vi "Create User Waveform.vi"(6 "Phase (0.0 deg)":dbl[](array[numeric])=[0.0, 0.0, 0.0, 0.0, 0.0, 0.0, 0.0, 0.0, 0.0, 0.0, 0.0, 0.0, 0.0, 0.0, 0.0, 0.0, 0.0, 0.0, 0.0, 0.0, 0.0, 0.0, 0.0, 0.0, 0.0, 0.0, 0.0, 0.0, 0.0, 0.0, 0.0, 0.0, 0.0, 0.0, 0.0, 0.0, 0.0, 0.0, 0.0, 0.0] min=0.0 max=359.7 format="%.1f", 7 "Memory Location (0)":u32 max=4, 8 "error in (no error)":errorcluster, 9 "Fundamental Frequency (60 Hz)":dbl=60.0 format="%#.2g", 10 "Weight Factor (0)":dbl[](array[numeric])=[0.0, 0.0, 0.0, 0.0, 0.0, 0.0, 0.0, 0.0, 0.0, 0.0, 0.0, 0.0, 0.0, 0.0, 0.0, 0.0, 0.0, 0.0, 0.0, 0.0, 0.0, 0.0, 0.0, 0.0, 0.0, 0.0, 0.0, 0.0, 0.0, 0.0, 0.0, 0.0, 0.0, 0.0, 0.0, 0.0, 0.0, 0.0, 0.0, 0.0] min=0.0 max=1.0 format="%#.6g", 11 "VISA resource name":refnum<visa-resource-name>) -> (0 "error out":errorcluster, 3 "VISA resource name out":refnum<visa-resource-name>)   [LabVIEW 2015, in "BK Precision 983X Series.lvlib"]
doc: "Configures output AC and DC voltage levels and frequency."
uses:
  <instrlib>/BK Precision 983X Series/BK Precision 983X Series.lvlib
panel:
  # "Hz"
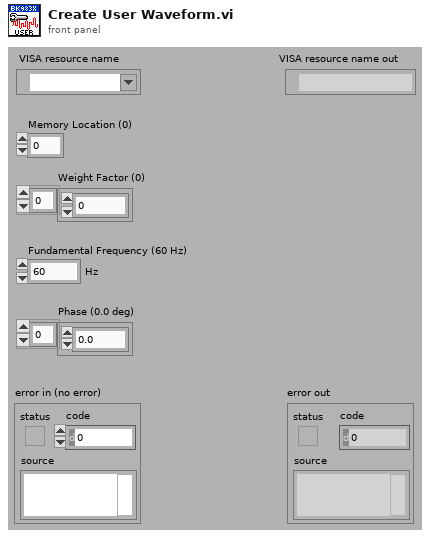
[diagram p1: front panel]
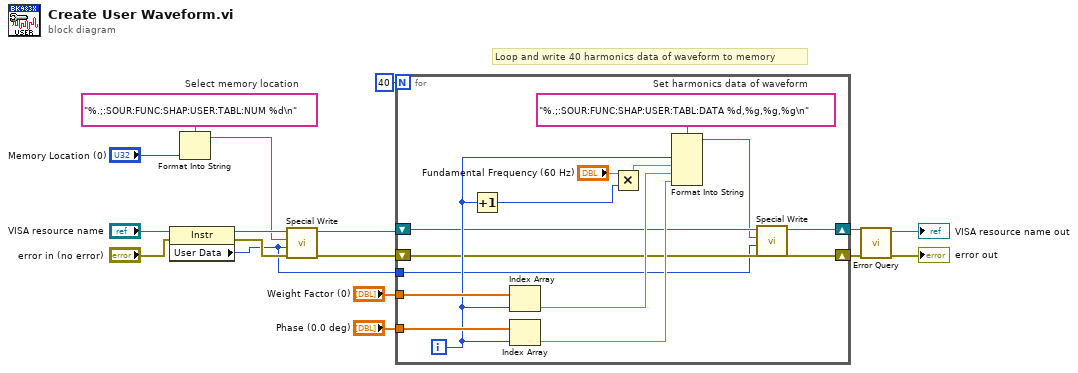
[diagram p0: block diagram]
diagram:
  w15 = "%.;:SOUR:FUNC:SHAP:USER:TABL:NUM %d\n"  # Select memory location
  # "Loop and write 40 harmonics data of waveform to memory"
  n1 = property class="Instr"(reference="VISA resource name", error in="error in (no error)") -> (reference out=w12:refnum<visa-resource-name>, error out=w11:errorcluster, "User Data"=w1:u32)
  n2 = Format Into String(format string=w15, "Memory Location (0)") -> (resulting string=w9:string)  [unwired: 2 in, 1 out]
  n3 = call <instrlib>:"Special Write.vi"("error in (no error)"=w11, "Delay (0 ms)"=w1, "Input String"=w9, "VISA resource name"=w12) -> ("error out"=w5:errorcluster, "VISA resource name out"=w4:refnum<visa-resource-name>)  [unwired: 6 in]
  n4 = for {
    N: 40 -> [_]
    tunnel: "Weight Factor (0)" -> [w28]
    tunnel: "Phase (0.0 deg)" -> [w27]
    tunnel: w1 -> [w19]
    shift-right: [w21] -> w3
    shift-left: w4 -> [w22]
    shift-right: [w20] -> w2
    shift-left: w5 -> [w23]
    i -> [w26]
    w32 = "%.;:SOUR:FUNC:SHAP:USER:TABL:DATA %d,%g,%g,%g\n"  # Set harmonics data of waveform
    n5 = Increment(x=w26) -> (x+1=w30:i32)
    n6 = Index Array(array=w28, index=w26) -> (element=w25:dbl)
    n7 = Index Array(array=w27, index=w26) -> (element=w24:dbl)
    n8 = Multiply(x="Fundamental Frequency (60 Hz)", y=w30) -> (x*y=w29:dbl)
    n9 = Format Into String(format string=w32, w26, w29, w25, w24) -> (resulting string=w18:string)  [unwired: 2 in, 1 out]
    n10 = call <instrlib>:"Special Write.vi"("error in (no error)"=w23, "Delay (0 ms)"=w19, "Input String"=w18, "VISA resource name"=w22) -> ("error out"=w20:errorcluster, "VISA resource name out"=w21:refnum<visa-resource-name>)  [unwired: 6 in]
  }
  n11 = call <instrlib>:"Error Query.vi"("error in (no error)"=w2, "VISA resource name"=w3) -> ("error out"=→"error out":errorcluster, "VISA resource name out"=→"VISA resource name out":refnum<visa-resource-name>)  [unwired: 6 in, 2 out]
